vi "initialise.vi"(6 "z":dbl[unit], 8 "error in (no error)":errorcluster, 9 "y":dbl[unit], 10 "x":dbl[unit], 11 "SpaceVector in":refnum<class "SpaceVector.lvclass">) -> (0 "error out":errorcluster, 3 "SpaceVector out":refnum<class "SpaceVector.lvclass">)   [LabVIEW 2010, in "SpaceVector.lvclass"]
uses:
  SpaceVector.lvclass
  arrays/space_vector_array.ctl
  SpaceVector.lvclass/SpaceVector.ctl
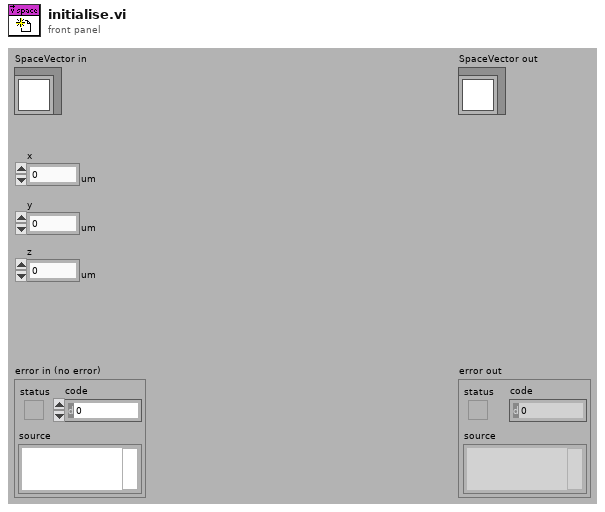
[diagram p1: front panel]
types:
  T1 = typedef "space_vector_array.ctl" = dbl[unit][]
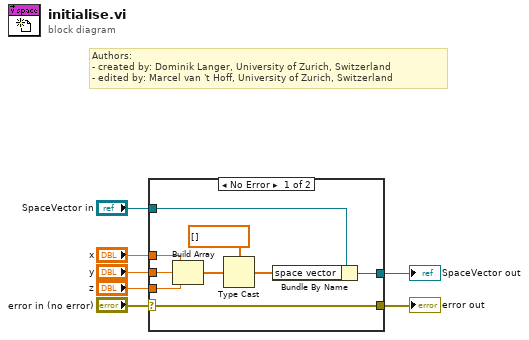
[diagram p0: block diagram]
diagram:
  # "Authors: \n- created by: Dominik Langer, University of Zurich, Switzerland\n- edited by: Marcel van 't Hoff, University of Zurich, Switzerland"
  n1 = case shown="No Error" "error in (no error)" {
    selector: "error in (no error)" -> [w16 w18]
    tunnel: [w16 w18] -> w6
    tunnel: [w14 w17] -> w4
    tunnel: "SpaceVector in" -> [w15 w17]
    tunnel: "x" -> [w13 _]
    tunnel: "y" -> [w12 _]
    tunnel: "z" -> [w11 _]
    frame No Error {
      n2 = Build Array(w13, w12, w11) -> (w10:dbl[unit][])
      n3 = Type Cast(type=T1 [] ("space vector"), x=w10) -> (*(type *) &x=w8:T1)
      n4 = Bundle By Name(cluster=w15, "space vector"=w8) -> (w14:refnum<class "SpaceVector.lvclass">)
    }
    frame Error {
    }
  }
  "error out" <- w6
  "SpaceVector out" <- w4
